vi "LogMissingElement).vi"(10 "Found?":bool, 11 "result string":string) -> ()   [LabVIEW 2013]
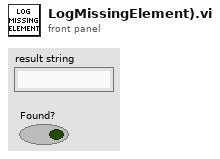
[diagram p1: front panel]
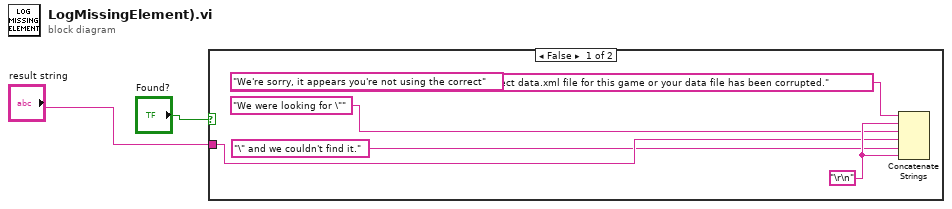
[diagram p0: block diagram]
diagram:
  n1 = case shown="False" "Found?" {
    tunnel: "result string" -> [w4 _]
    frame False {
      w7 = "\r\n"
      (unwired) "We're sorry, it appears you're not using the correct"
      n2 = Concatenate Strings("We're sorry, it appears you're wither not using the correct data.xml file for this game or your data file has been corrupted.", w7, "We were looking for \"", w4, "\" and we couldn't find it.", w7) -> ()  [unwired: 1 out]
    }
    frame True {
    }
  }
